vi "getValue.vi"(8 "error in (no error)":errorcluster, 11 "tBSONDocumentElement in":refnum<class "tBSONDocumentElement.lvclass">) -> (0 "error out":errorcluster, 2 "Value":refnum<class "tBSONDocument.lvclass">, 3 "tBSONDocumentElement out":refnum<class "tBSONDocumentElement.lvclass">)   [LabVIEW 2013, in "BSON.lvlib" / "tBSONDocumentElement.lvclass"]
uses:
  tBSONDocumentElement.lvclass
  tBSONDocument/tBSONDocument.lvclass
  tBSONDocumentElement.lvclass/tBSONDocumentElement.ctl
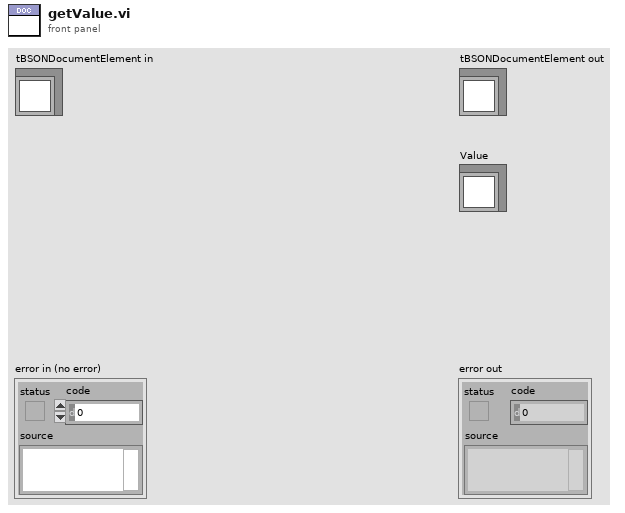
[diagram p1: front panel]
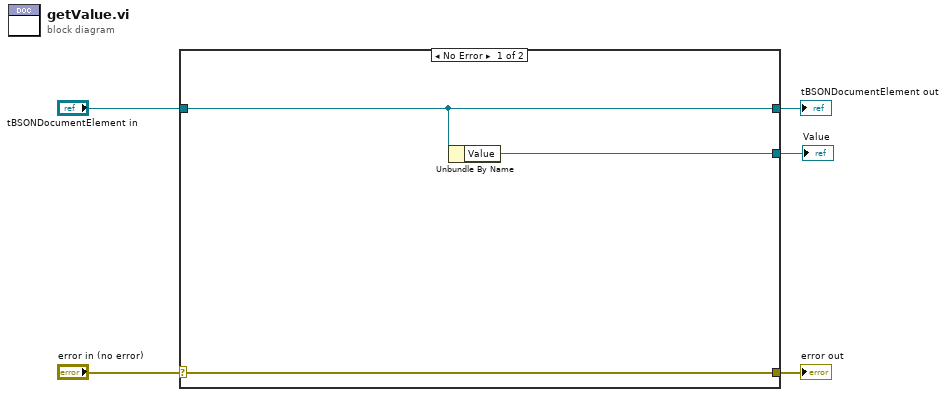
[diagram p0: block diagram]
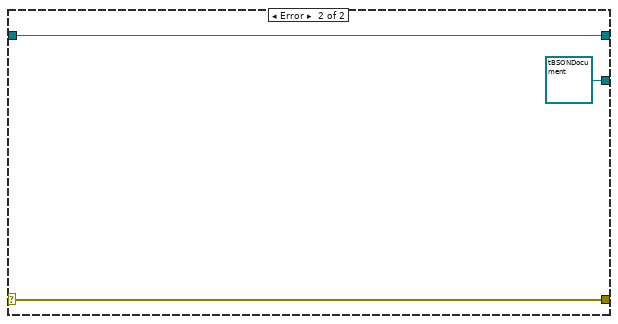
[diagram p2: hidden frame]
diagram:
  n1 = case shown="No Error" "error in (no error)" {
    selector: "error in (no error)" -> [w8 w11]
    tunnel: [w8 w11] -> w4
    tunnel: [w7 w10] -> w2
    tunnel: "tBSONDocumentElement in" -> [w7 w10]
    tunnel: [w6 refnum<class "tBSONDocument.lvclass"> refnum ("Value")] -> w1
    frame No Error {
      n2 = Unbundle By Name(w7) -> ("Value"=w6:refnum<class "tBSONDocument.lvclass">)
    }
    frame Error {
    }
  }
  "error out" <- w4
  "tBSONDocumentElement out" <- w2
  "Value" <- w1
